vi "Step global.vi"() -> ()   [LabVIEW 2014]
uses:
  Control/Step name enum.ctl
panel:
  in  "Step cluster":T2={"Step number"=0, "Step Name"="", "Step name enum"=enum."Init NI", "Start condition 1 name"="", "Start condition 1 comparator"="", "Start condition 1 value"=0.0, "Start condition 2 name"="", "Start condition 2 comparator"="", "Start condition 2 value"=0.0, "Start condition 3 name"="", "Start condition 3 comparator"="", "Start condition 3 value"=0.0, "End condition 1 name"="", "End condition 1 comparator"="", "End condition 1 value"=0.0, "End condition 2 name"="", "End condition 2 comparator"="", "End condition 2 value"=0.0, "End condition 3 name"="", "End condition 3 comparator"="", "End condition 3 value"=0.0, "Constant condition 1 name"="", "Constant condition 1 comparator"="", "Constant condition 1 value"=0.0, "Constant condition 2 name"="", "Constant condition 2 comparator"="", "Constant condition 2 value"=0.0, "Constant condition 3 name"="", "Constant condition 3 comparator"="", "Constant condition 3 value"=0.0, "Duration, mS"=0.0, "Max Duration, mS"=0.0}
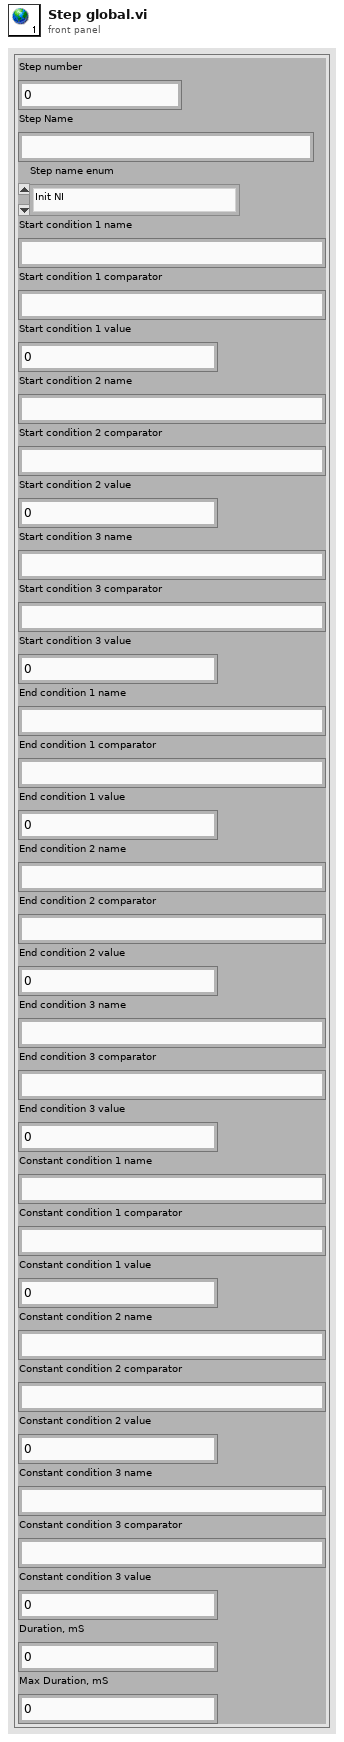
[diagram p1: front panel]
types:
  T1 = typedef "Step name enum.ctl" = enum16{"Default", "Idle", "Init Ard", "Init SM", "Init NI", "Run", "Close"}
  T2 = cluster{"Step number":i32, "Step Name":string, "Step name enum":T1, "Start condition 1 name":string, "Start condition 1 comparator":string, "Start condition 1 value":dbl, "Start condition 2 name":string, "Start condition 2 comparator":string, "Start condition 2 value":dbl, "Start condition 3 name":string, "Start condition 3 comparator":string, "Start condition 3 value":dbl, "End condition 1 name":string, "End condition 1 comparator":string, "End condition 1 value":dbl, "End condition 2 name":string, "End condition 2 comparator":string, "End condition 2 value":dbl, "End condition 3 name":string, "End condition 3 comparator":string, "End condition 3 value":dbl, "Constant condition 1 name":string, "Constant condition 1 comparator":string, "Constant condition 1 value":dbl, "Constant condition 2 name":string, "Constant condition 2 comparator":string, "Constant condition 2 value":dbl, "Constant condition 3 name":string, "Constant condition 3 comparator":string, "Constant condition 3 value":dbl, "Duration, mS":dbl, "Max Duration, mS":dbl}
diagram:
